vi "testAppBuilder_rt.vi"() -> ()   [LabVIEW 2014]
uses:
  <vilib>/FPGAPlugInAG/myRIO-1900/niLvFpga_Open_myRIO-1900.vi
  <vilib>/rvi/interface/common/dynamic/niFpgaDynamicAddResources.vi
  <vilib>/Utility/error.llb/Error Cluster From Error Code.vi
  <vilib>/rvi/errors/niLvFpgaAdjustHostInterfaceError.vi
  <vilib>/FPGAPlugInAG/Dynamic/niLvFpga_Close_Dynamic.vi
  <vilib>/rvi/interface/nirviOpenFPGA/nirviOpenFPGA.xnode
  testAppBuilder_fpga_build.lvbitx
  testAppBuilder_fpga.vi
  <vilib>/rvi/interface/nirviReadWriteControl/nirviReadWriteControl.xnode
  <vilib>/rvi/interface/nirviCloseFPGA/nirviCloseFPGA.xnode
  NiFpgaLv.dll
  <vilib>/rvi/interface/Simulation/niFpgaSimulationCallBeginRW.vi
panel:
  in  "stop":bool
  out "output_num":i16
  in  "input_num":i16=4
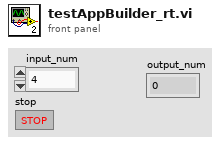
[diagram p1: front panel]
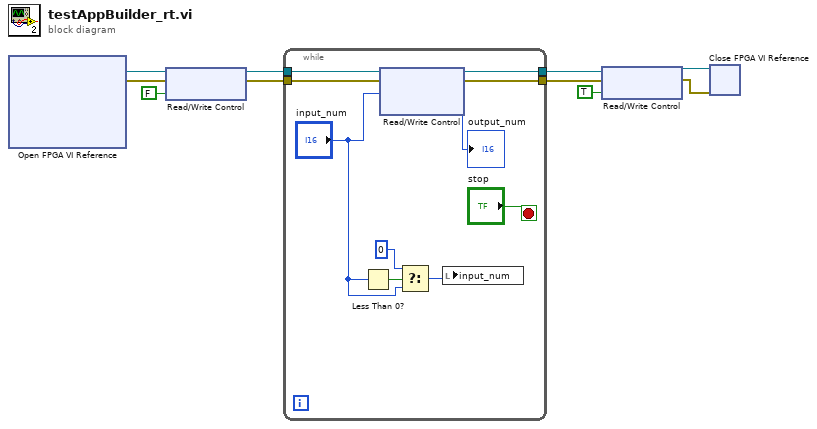
[diagram p0: block diagram]
diagram:
  n1 = xnode "Open FPGA VI Reference"() -> ("FPGA VI Reference Out"=w10:refnum<k20>, "error out"=w9:errorcluster)  [unwired: 2 in]
  n2 = xnode "Read/Write Control"("FPGA VI Reference In"=w10, "error in"=w9, "input_STOP"=FALSE) -> ("FPGA VI Reference Out"=w6:refnum<k20>, "error out"=w7:errorcluster)
  n3 = while {
    tunnel: w7 -> [w20]
    tunnel: w6 -> [w19]
    tunnel: [w16] -> w5
    tunnel: [w15] -> w4
    stop <- "stop" stop-if-true
    n4 = Less Than 0?(x="input_num") -> (x < 0?=w14:bool)
    n5 = xnode "Read/Write Control"("FPGA VI Reference In"=w19, "error in"=w20, "input_num"="input_num") -> ("FPGA VI Reference Out"=w16:refnum<k20>, "error out"=w15:errorcluster, "output_num"=→"output_num":i16)
    n6 = Select(t=i16 0, s=w14, f="input_num") -> (s? t:f=w11:i16)
    n7 = local write "input_num"(w11) -> ()
  }
  n8 = xnode "Read/Write Control"("FPGA VI Reference In"=w5, "error in"=w4, "input_STOP"=TRUE) -> ("FPGA VI Reference Out"=w2:refnum<k20>, "error out"=w1:errorcluster)
  n9 = xnode "Close FPGA VI Reference"("FPGA VI Reference In"=w2, "error in"=w1) -> ()  [unwired: 1 out]
